vi "Handle Messages.vi"(10 "Current Msgs":string[](array[string]), 11 "nData in":refnum<class "SOAP Data.lvclass">) -> (3 "nData out":refnum<class "SOAP Data.lvclass">)   [LabVIEW 2017, in "Controller.lvlib" / "SOAP Data.lvclass"]
uses:
  SOAP Data.lvclass
  SOAP Data.lvclass/SOAP Data.ctl
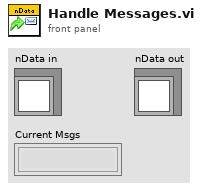
[diagram p1: front panel]
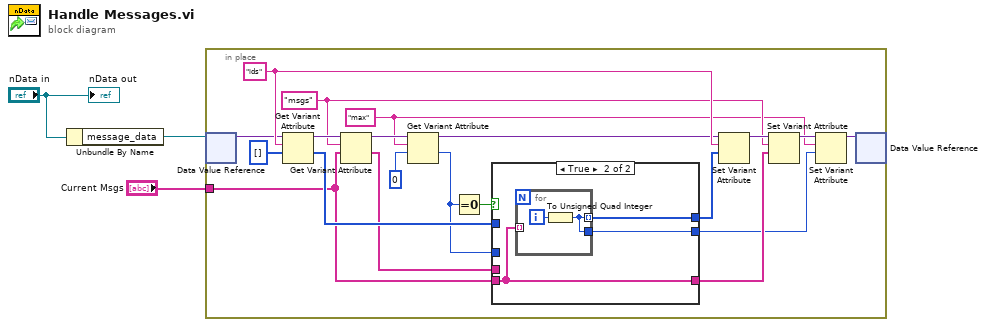
[diagram p0: block diagram]
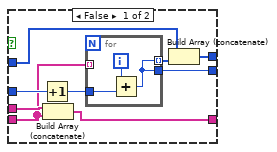
[diagram p2: hidden frame]
diagram:
  n1 = Unbundle By Name("nData in") -> ("message_data"=w2:refnum<data-value>)
  n2 = in-place {
    in-place-border: "Current Msgs" -> [w19]
    w8 = "max" ("name")
    w16 = "msgs" ("name")
    w21 = "ids" ("name")
    n3 = in-place-dvr #1(w2) -> (w6:variant)  [unwired: 1 out]
    n4 = Get Variant Attribute(Variant=w6, name=w21, default value (empty Variant)=u64[] []) -> (duplicate Variant=w20:variant, value=w22:u64[])  [unwired: 1 in, 2 out]
    n5 = Get Variant Attribute(Variant=w20, name=w16, default value (empty Variant)=w19) -> (duplicate Variant=w13:variant, value=w18:string[])  [unwired: 1 in, 2 out]
    n6 = Get Variant Attribute(Variant=w13, name=w8, default value (empty Variant)=u64 0) -> (duplicate Variant=w11:variant, value=w9:u64)  [unwired: 1 in, 2 out]
    n7 = Equal To 0?(x=w9) -> (x = 0?=w10:bool)
    n8 = case shown="True" w10 {
      tunnel: w22 -> [w26 _]
      tunnel: [w24 w38] -> w4
      tunnel: w19 -> [w27 w37]
      tunnel: [w28 w37] -> w15
      tunnel: w18 -> [w29 _]
      tunnel: w9 -> [w32 _]
      tunnel: [w30 w36] -> w7
      frame False {
        n9 = Increment(x=w32) -> (x+1=w31:u64)
        n10 = Build Array (concatenate)(w29, w27) -> (w28:string[])
        n11 = for {
          tunnel: w31 -> [w34]
          tunnel: [w33] -> w25 mode=indexing
          tunnel: [w33] -> w30
          tunnel: w27 -> [_] mode=indexing
          i -> [w35]
          n12 = Add(x=w35, y=w34) -> (x+y=w33:u64)
        }
        n13 = Build Array (concatenate)(w26, w25) -> (w24:u64[])
      }
      frame True {
        n14 = for {
          tunnel: [w39] -> w38 mode=indexing
          tunnel: w37 -> [_] mode=indexing
          tunnel: [w39] -> w36
          i -> [w40]
          n15 = To Unsigned Quad Integer(1:w40) -> (0:w39:u64)
        }
      }
    }
    n16 = Set Variant Attribute(Variant=w11, name=w21, value=w4) -> (Variant out=w17:variant)  [unwired: 1 in, 2 out]
    n17 = Set Variant Attribute(Variant=w17, name=w16, value=w15) -> (Variant out=w14:variant)  [unwired: 1 in, 2 out]
    n18 = Set Variant Attribute(Variant=w14, name=w8, value=w7) -> (Variant out=w5:variant)  [unwired: 1 in, 2 out]
    n19 = in-place-dvr #1(w5) -> ()  [unwired: 2 out]
  }
  "nData out" <- "nData in"
